vi "ICRA2024测试椭圆分裂0902修改版.vi"() -> ()   [LabVIEW 2018]
doc: "Demonstrates the use of the Network Streams functions to send LED status to the myRIO target."
uses:
  <vilib>/vision/Contour.llb/IMAQ Contour Curve Extraction.ctl
  <vilib>/ErrorRing/Error Ring.xnode
  <vilib>/vision/NI_Vision_Development_Module.lvlib
panel:
  out "数据总":dbl[][](array[numeric])
  out "pitch angle2":dbl[](array[numeric])
  out "pitch angle1":sgl[](array[numeric])
  out "direction angle":sgl[](array[numeric])
  out "磁场ratio":sgl[](array[numeric])
  out "磁场频率":sgl[](array[numeric])
  out "T":i32[](array[numeric])
  out "ratio":dbl[](array[numeric])
  out "长度2":i32[](array[numeric])
  out "宽度":i32[](array[numeric])
  in  "数据记录":bool
  out "ratio":dbl
  out "长度2":i32
  out "宽度":i32
  out "Y Bottom":i32
  out "X Right":i32
  out "Y Top":i32
  out "X Left":i32
  in  "Rectangle 3":T1={"Left"=500, "Top"=800, "Right"=800, "Bottom"=1100}
  in  "Rectangle 2":T1={"Left"=500, "Top"=500, "Right"=800, "Bottom"=600}
  in  "Rectangle":T1={"Left"=500, "Top"=0, "Right"=800, "Bottom"=300}
  in  "Search Rect (entire image)":T2={"Left"=200, "Top"=120, "Right"=2000, "Bottom"=1920, "Rotation"=0.0} {"Rotation" format="%.2f"; "Left" scale=0.0..1024.0; "Right" scale=0.0..1024.0}
  out "长度":dbl
  out "备用的椭圆角度":sgl
  out "Image 9":T3(plugin-control)
  in  "Search Direction":T4(ring)
  in  "Contour Selection":T5(ring)
  in  "Number of Erosion":i32=10
  in  "椭圆磁场开关":bool=TRUE
  out "Image 7":T3(plugin-control)
  out "Ellipse":T6 {"Center"."Y" format="%.2f"; "Center"."X" format="%.2f"}
  out "Image 5":T3(plugin-control)
  in  "Contour Points Settings":T7={"Overlay?"=FALSE, "Color"=16711680, "Width"=1, "Maintain Width?"=TRUE}
  in  "Contour Equation Settings":T7={"Overlay?"=TRUE, "Color"=3381759, "Width"=1, "Maintain Width?"=TRUE}
  out "ROI Descriptor Out":T8 {"Contours"."Type" items=["No Selection", "Point", "Line", "Rectangle", "Oval", "Polygon", "Freehand Region", "Annulus", "Unused2", "Unused3", "Broken Line", "Freehand Line", "Rotated Rectangle"]}
  in  "Curve Extraction":T9={"Extraction Mode"=0, "Edge Threshold"=75, "Edge Filter Size"=1, "Min Length"=25, "Search Step Size"=15, "Max Endpoint Gap"=10, "Subpixel"=TRUE} {"Extraction Mode" items=["Normal", "Uniform Regions"]; "Edge Filter Size" items=["Fine", "Normal", "Contour Tracing"]; "Max Endpoint Gap" min=0; "Search Step Size" min=1 max=255 step=1; "Min Length" min=0; "Edge Threshold" min=1 max=350 step=1}
  out "Image 4":T3(plugin-control)
  out "Image":T3(plugin-control)
  in  "Acquisition Control::Acquisition Frame Rate":dbl=19.50304412841797 min=1.4211589097976685 max=44.94382095336914
  out "Stopped":bool
  in  "Stop (F) 2":bool caption="Stop (F)"
  out "Objects 2":T10(array[cluster]) {"Aspect Ratio" format="%.2f"; "Orientation" format="%.2f"; "Area" format="%.2f"; "Object Center"."Y" format="%.2f"; "Object Center"."X" format="%.2f"}
  in  "Settings 2":T11={"Objects"=0, "Threshold"=128, "Reject Border"=FALSE, "Fill Holes"=FALSE, "Min Object Size"=TRUE, "Min Size"=20000, "Max Object Size"=FALSE, "Max Size"=100, "Show Search Area"=FALSE, "Show Center"=TRUE, "Show Bounding Box"=TRUE} {"Objects" items=["Bright Objects", "Dark Objects"]; "Threshold" min=1 max=999999999 step=1; "Max Size" min=1 max=999999999 step=1; "Min Size" min=1 max=999999999 step=1}
  in  "Range 2":cluster{"Lower value":sgl, "Upper value":sgl}={"Lower value"=0.0, "Upper value"=230.0} {"Upper value" format="%.2f"; "Lower value" format="%.2f"}
  in  "Pause":bool
  out "Array":dbl[](array[numeric])
  in  "Parameter Settings":T12(tab)=enum."Ribbon Oscillating Field" caption="Field Types"
  in  "fg":dbl
  in  "pg":dbl
  in  "dg":dbl
  in  "Ag":dbl
  in  "AoOF":dbl
  in  "fo":sgl
  in  "do":sgl
  in  "oo":sgl
  in  "po":sgl
  in  "cc":sgl
  in  "pc":sgl
  in  "wc":sgl
  in  "dc":sgl
  in  "Ac":dbl
  in  "pr":sgl
  in  "Ar":dbl=8.0
  in  "wr":sgl=18.0
  in  "dr":sgl
  in  "Dis phase step":dbl
  in  "Dis phase frequency (Hz)":dbl
  in  "Dis tumbling frequency (Hz)":dbl
  in  "Dis strength(mT)":dbl
  in  "Swa strength (mT)":dbl
  in  "Swa frequency (Hz)":dbl
  in  "Swa pitch angle (deg)":dbl
  in  "Swa direction angle (deg)":dbl
  in  "Swa ratio":dbl=1.0
  in  "Pitch Angle (rotating around Constant, deg)":dbl
  in  "Ratio (A/C)":sgl=3.0
  in  "Direction Angle (deg)":sgl=90.0
  in  "Pitch Angle (rotating around Origin, deg)":sgl
  in  "Frequency (Hz)":sgl=6.0
  in  "Strength (mT)":dbl=3.0
  in  "Ar 2":dbl=5.0 caption="Ar"
  in  "ratio":sgl=1.0
  in  "运动方向":sgl
  in  "长轴方向":sgl
  in  "wr  2":sgl=8.0
  in  "速度大小":sgl
  out "Angle":dbl
  out "aspect ratio":dbl
  out "时间":i32
  out "Numeric 5":i32
  in  "Stop":bool
  out "error out":errorcluster
  in  "Target IP Address":string="172.22.11.2"
  # "Overview: Magnetic field calculation, and send parameters to myRIO\nInstructions:\n1. Verify the value of Target IP Address. Set Visa resource name.\n2. Ensure RT Main.vi is already running. \n3. Run this VI. Set parameters of magnetic field."
  # "Strength (mT)"
  # "Pitch Angle (deg)"
  # "Direction Angle (deg)"
  # "Frequency (Hz)"
  # "Strength (mT)"
  # "Oscilation Frequency (Hz)"
  # "Oscilation Angle (deg)"
  # "Pitch Angle (deg)"
  # "Direction Angle (deg)"
  # "Strength (mT)"
  # "Frequency (Hz)"
  # "Pitch Angle (deg)"
  # "Direction Angle (deg)"
  # "Conical Angle (deg)"
  # "Strength (mT)"
  # "Frequency (Hz)"
  # "Pitch Angle (deg)"
  # "Direction Angle (deg)"
  # "Strength (mT)"
  # "Tumbling Frequency (Hz)"
  # "Phase Frequency (Hz)"
  # "Phase Step"
  # "Strength (mT)"
  # "Frequency (Hz)"
  # "Pitch Angle (deg)"
  # "Direction Angle (deg)"
  # "Ratio"
  # "Strength (mT)"
  # "Frequency (Hz)"
  # "Ratio (A/C)"
  # "Direction Angle (deg)"
  # "Pitch Angle (rotating around Origin, deg)"
  # "Pitch Angle (rotating around Constant, deg)"
  # "Strength (mT)"
  # "Frequency (Hz)"
  # "Pitch Angle  (deg)"
  # "longaxis"
  # "Direction Angle (deg)"
  # "ratio (l/s)"
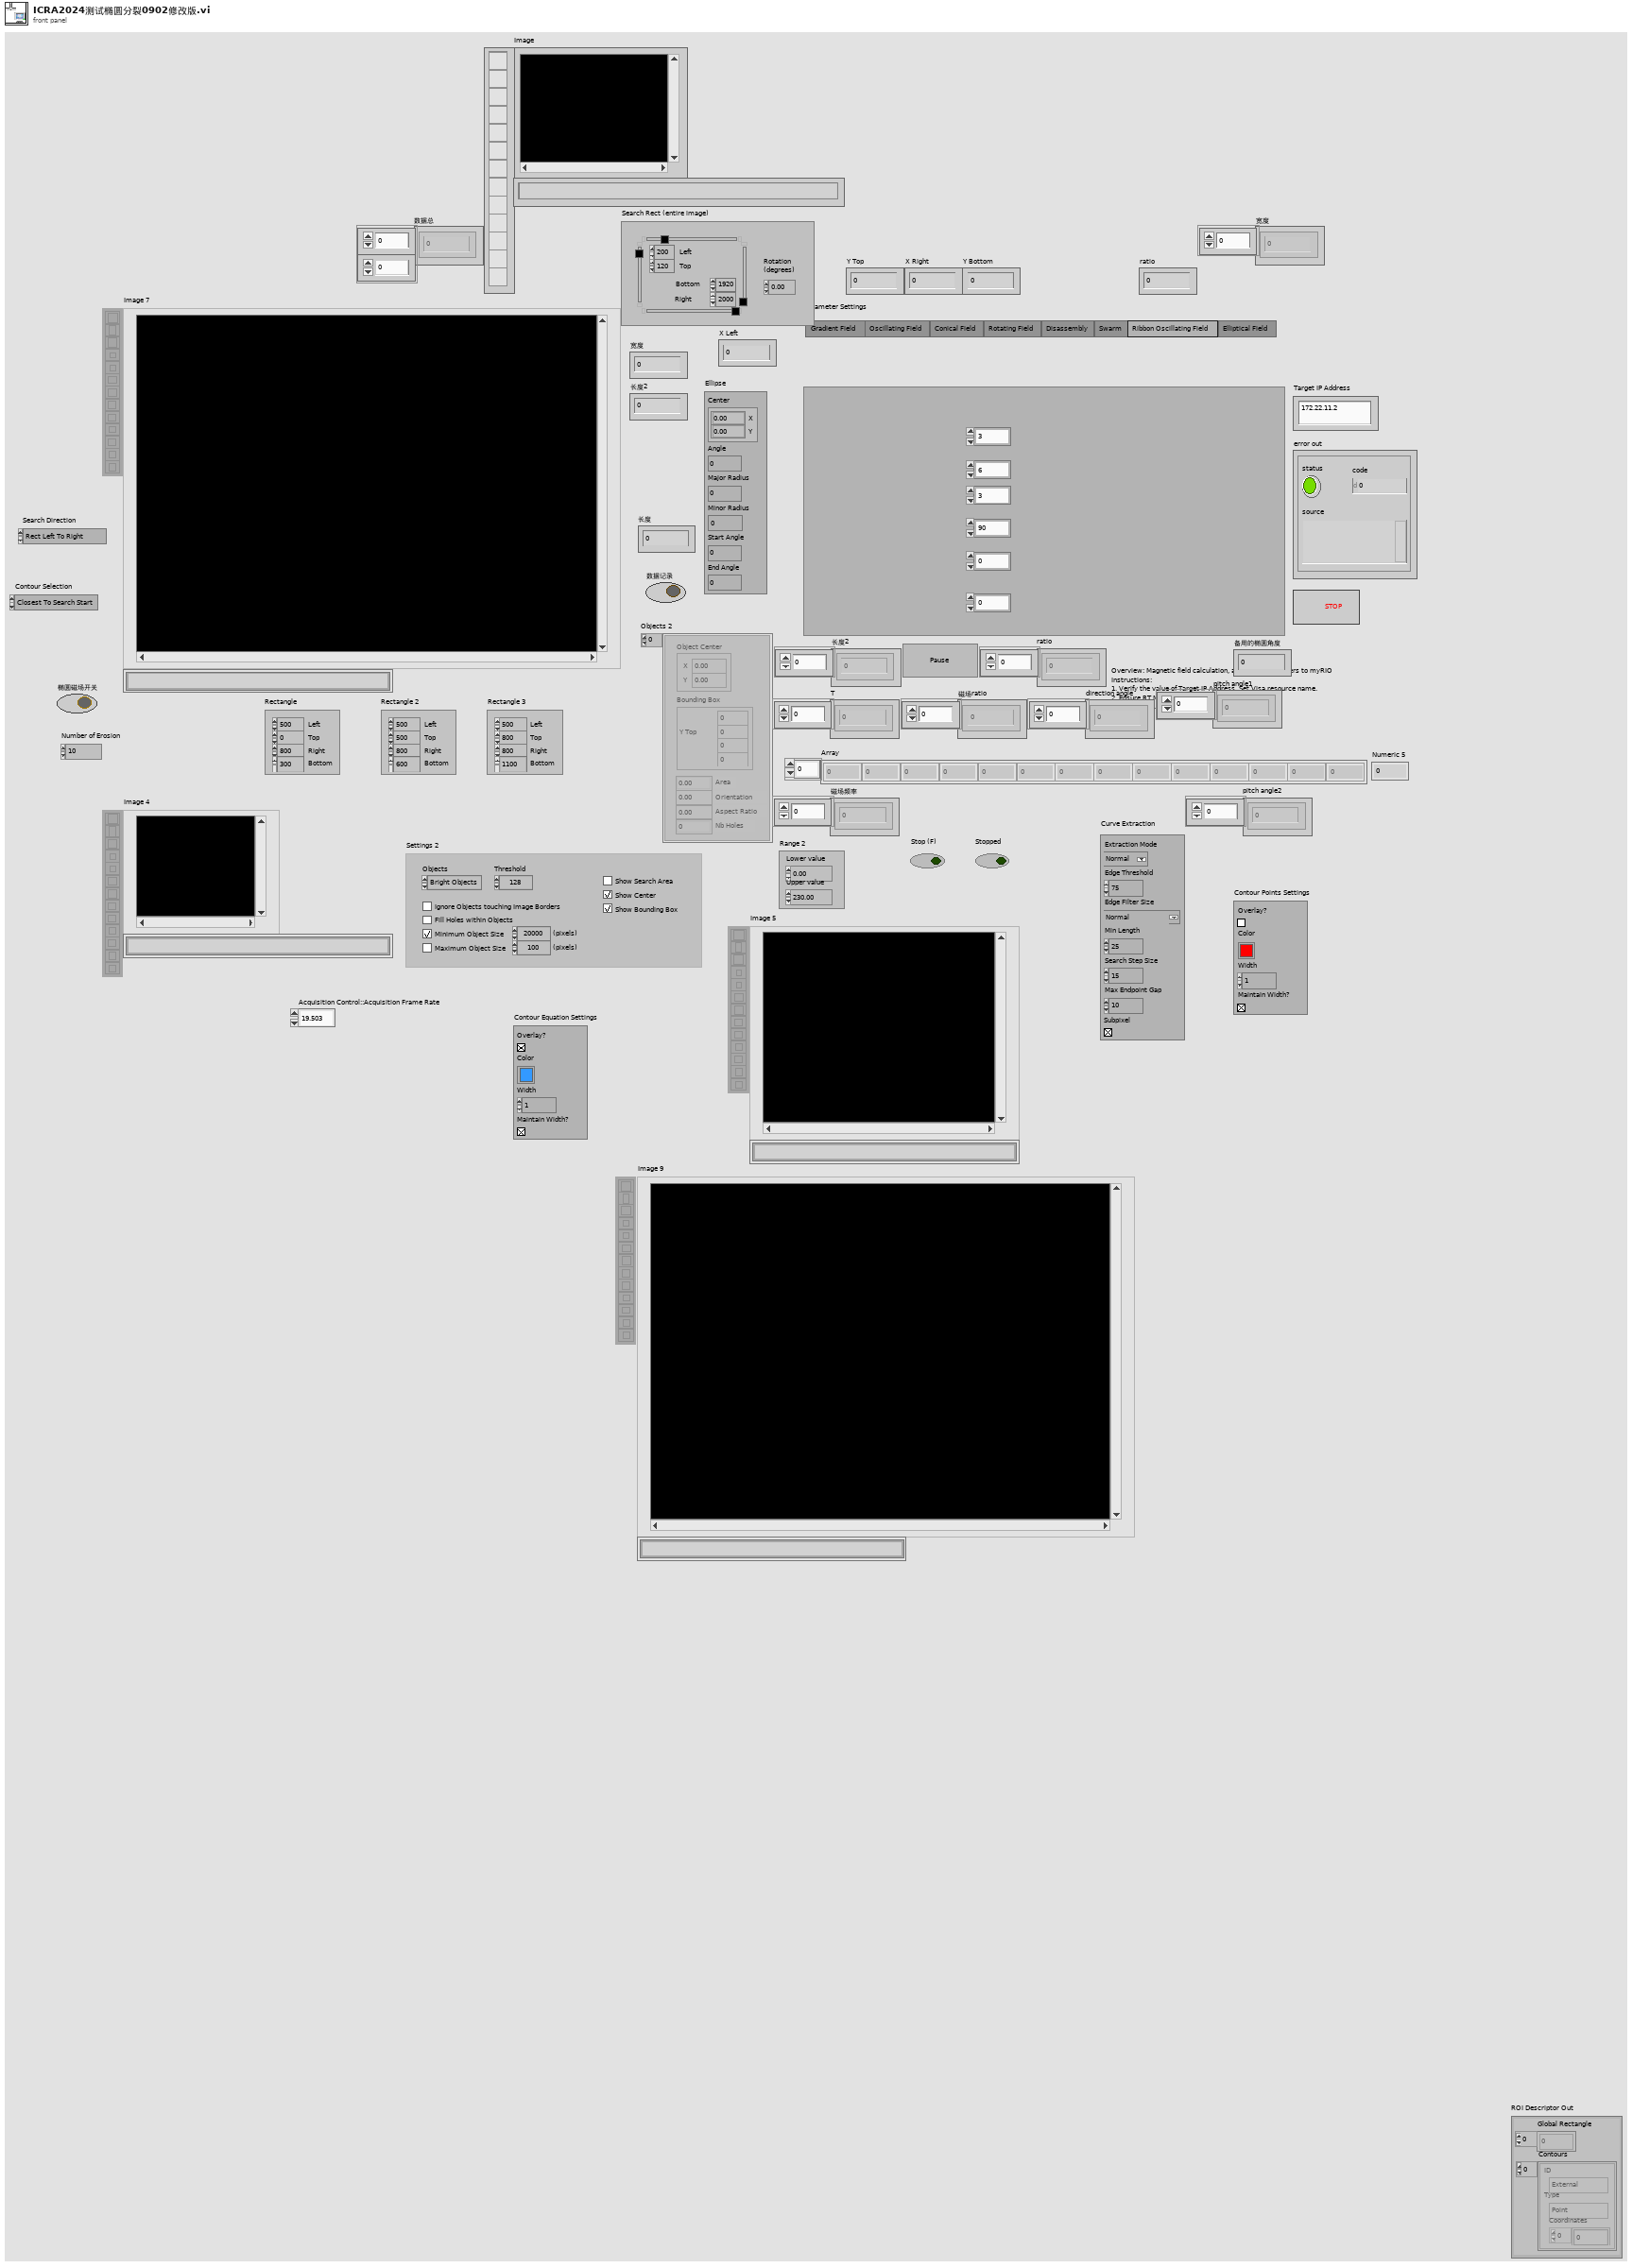
[diagram p1: front panel]
types:
  T1 = cluster{"Left":i32, "Top":i32, "Right":i32, "Bottom":i32}
  T2 = typedef "IMAQ Rectangle" = cluster{"Left":i32, "Top":i32, "Right":i32, "Bottom":i32, "Rotation":dbl}
  T3 = typedef "IMAQ Image.ctl" = refnum<image>
  T4 = enum16{"Rect Left To Right", "Rect Right To Left", "Rect Top To Bottom", "Rect Bottom To Top", "Annulus Inner To Outer", "Annulus Outer To Inner", "Annulus Start Angle To End Angle", "Annulus End Angle To Start Angle"}
  T5 = enum16{"Closest To Search Start", "Maximum Length", "Strongest Mean Gradient Change"}
  T6 = cluster{"Center":cluster{"X":sgl, "Y":sgl}, "Angle":dbl, "Major Radius":dbl, "Minor Radius":dbl, "Start Angle":dbl, "End Angle":dbl}
  T7 = cluster{"Overlay?":bool, "Color":u32, "Width":u32, "Maintain Width?":bool}
  T8 = typedef "ROI Descriptor" = cluster{"Global Rectangle":i32[], "Contours":cluster{"ID":enum32{"External", "Internal"}, "Type":u32, "Coordinates":i32[]}[]}
  T9 = typedef "IMAQ Contour Curve Extraction.ctl" = cluster{"Extraction Mode":u32, "Edge Threshold":i32, "Edge Filter Size":u32, "Min Length":i32, "Search Step Size":i32, "Max Endpoint Gap":i32, "Subpixel":bool}
  T10 = cluster{"Object Center":cluster{"X":sgl, "Y":sgl}, "Bounding Box":cluster{"X Left":i32, "Y Top":i32, "X Right":i32, "Y Bottom":i32}, "Area":sgl, "Orientation":sgl, "Aspect Ratio":sgl, "Nb Holes":i32}[]
  T11 = cluster{"Objects":u16, "Threshold":i32, "Reject Border":bool, "Fill Holes":bool, "Min Object Size":bool, "Min Size":i32, "Max Object Size":bool, "Max Size":i32, "Show Search Area":bool, "Show Center":bool, "Show Bounding Box":bool}
  T12 = enum32{"Gradient Field ", "Oscillating Field", "Conical Field", "Rotating Field", "Disassembly", "Swarm", "Ribbon Oscillating Field", "Elliptical Field"}
  T13 = enum32{"AutoM", "Close", "Dilate", "Erode", "Gradient", "Gradient in", "Gradient out", "HitMiss", "Open", "PClose", "POpen", "Thick", "Thin"}
  T14 = typedef "Image Type" = u32
  T15 = cluster{"Objects[0]":cluster{"Object Center":cluster{"X":sgl, "Y":sgl}, "Bounding Box":cluster{"X Left":i32, "Y Top":i32, "X Right":i32, "Y Bottom":i32}, "Area":sgl, "Orientation":sgl, "Aspect Ratio":sgl, "Nb Holes":i32}, "Objects[1]":cluster{"Object Center":cluster{"X":sgl, "Y":sgl}, "Bounding Box":cluster{"X Left":i32, "Y Top":i32, "X Right":i32, "Y Bottom":i32}, "Area":sgl, "Orientation":sgl, "Aspect Ratio":sgl, "Nb Holes":i32}, "Objects[2]":cluster{"Object Center":cluster{"X":sgl, "Y":sgl}, "Bounding Box":cluster{"X Left":i32, "Y Top":i32, "X Right":i32, "Y Bottom":i32}, "Area":sgl, "Orientation":sgl, "Aspect Ratio":sgl, "Nb Holes":i32}, "Objects[3]":cluster{"Object Center":cluster{"X":sgl, "Y":sgl}, "Bounding Box":cluster{"X Left":i32, "Y Top":i32, "X Right":i32, "Y Bottom":i32}, "Area":sgl, "Orientation":sgl, "Aspect Ratio":sgl, "Nb Holes":i32}, "Objects[4]":cluster{"Object Center":cluster{"X":sgl, "Y":sgl}, "Bounding Box":cluster{"X Left":i32, "Y Top":i32, "X Right":i32, "Y Bottom":i32}, "Area":sgl, "Orientation":sgl, "Aspect Ratio":sgl, "Nb Holes":i32}, "Objects[5]":cluster{"Object Center":cluster{"X":sgl, "Y":sgl}, "Bounding Box":cluster{"X Left":i32, "Y Top":i32, "X Right":i32, "Y Bottom":i32}, "Area":sgl, "Orientation":sgl, "Aspect Ratio":sgl, "Nb Holes":i32}, "Objects[6]":cluster{"Object Center":cluster{"X":sgl, "Y":sgl}, "Bounding Box":cluster{"X Left":i32, "Y Top":i32, "X Right":i32, "Y Bottom":i32}, "Area":sgl, "Orientation":sgl, "Aspect Ratio":sgl, "Nb Holes":i32}, "Objects[7]":cluster{"Object Center":cluster{"X":sgl, "Y":sgl}, "Bounding Box":cluster{"X Left":i32, "Y Top":i32, "X Right":i32, "Y Bottom":i32}, "Area":sgl, "Orientation":sgl, "Aspect Ratio":sgl, "Nb Holes":i32}, "Objects[8]":cluster{"Object Center":cluster{"X":sgl, "Y":sgl}, "Bounding Box":cluster{"X Left":i32, "Y Top":i32, "X Right":i32, "Y Bottom":i32}, "Area":sgl, "Orientation":sgl, "Aspect Ratio":sgl, "Nb Holes":i32}}
  T16 = cluster{"Object Center":cluster{"X":sgl, "Y":sgl}, "Bounding Box":cluster{"X Left":i32, "Y Top":i32, "X Right":i32, "Y Bottom":i32}, "Area":sgl, "Orientation":sgl, "Aspect Ratio":sgl, "Nb Holes":i32}
  T17 = cluster{"X Left":i32, "Y Top":i32, "X Right":i32, "Y Bottom":i32}
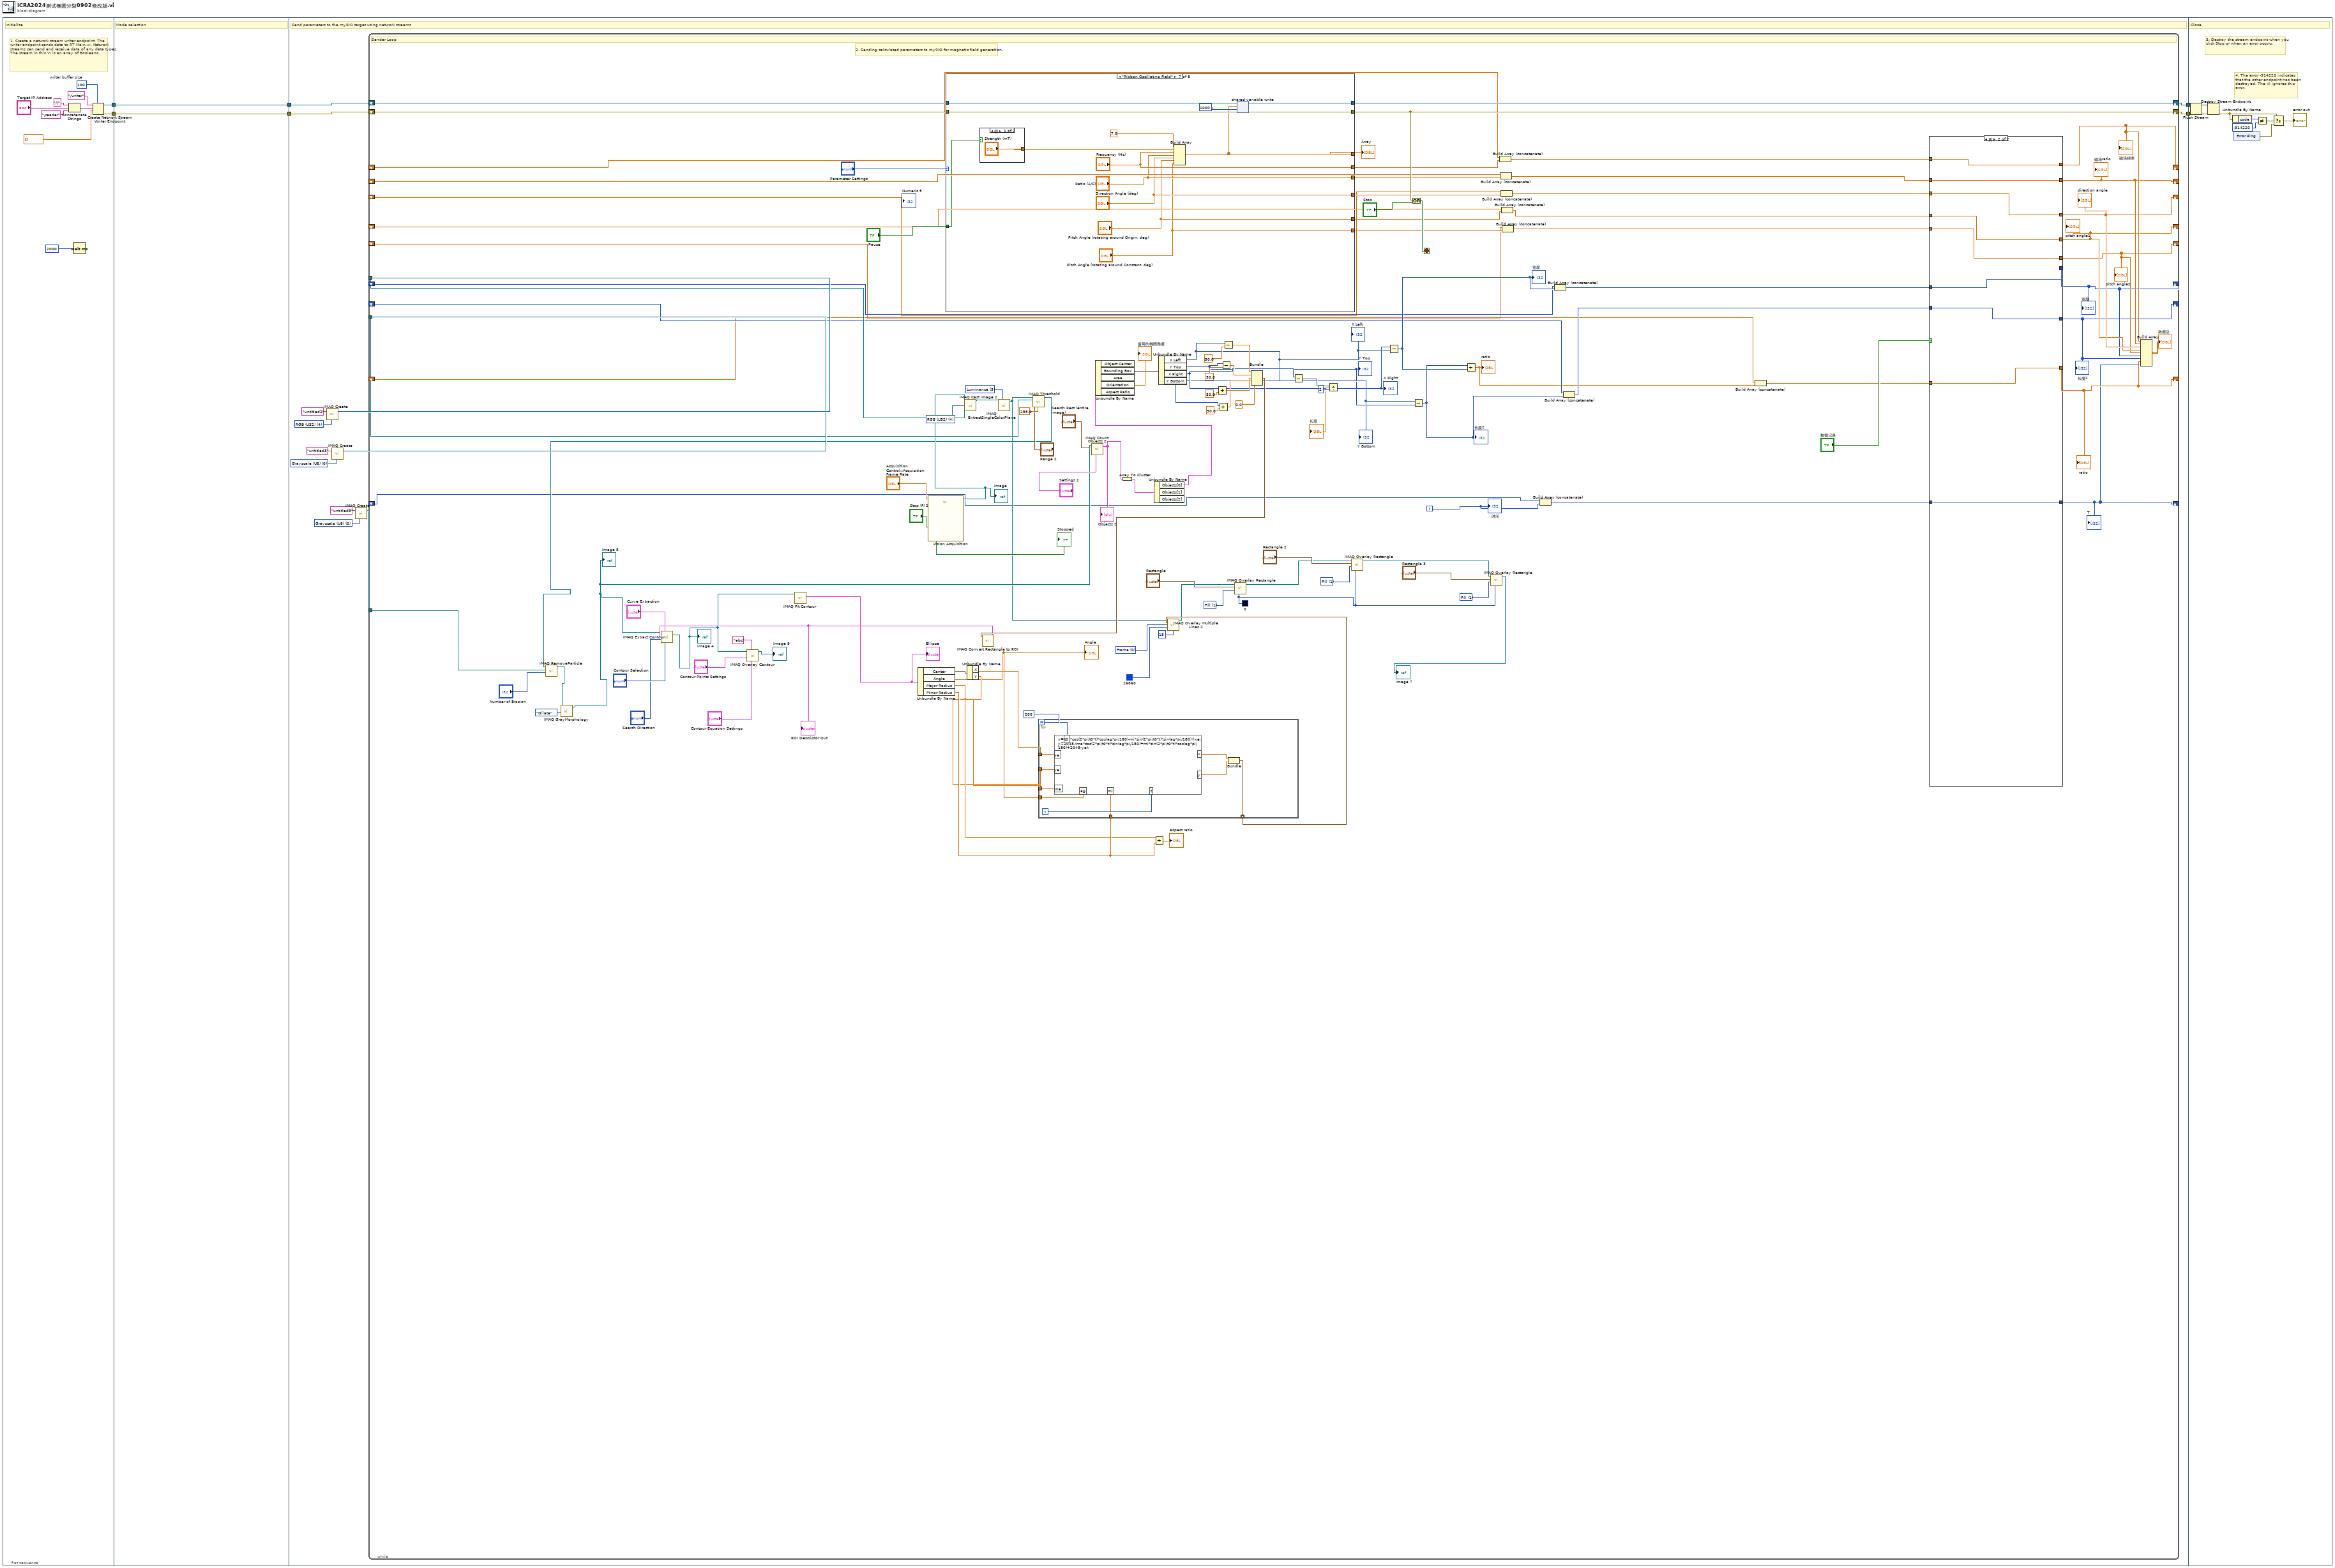
[diagram p0: block diagram]
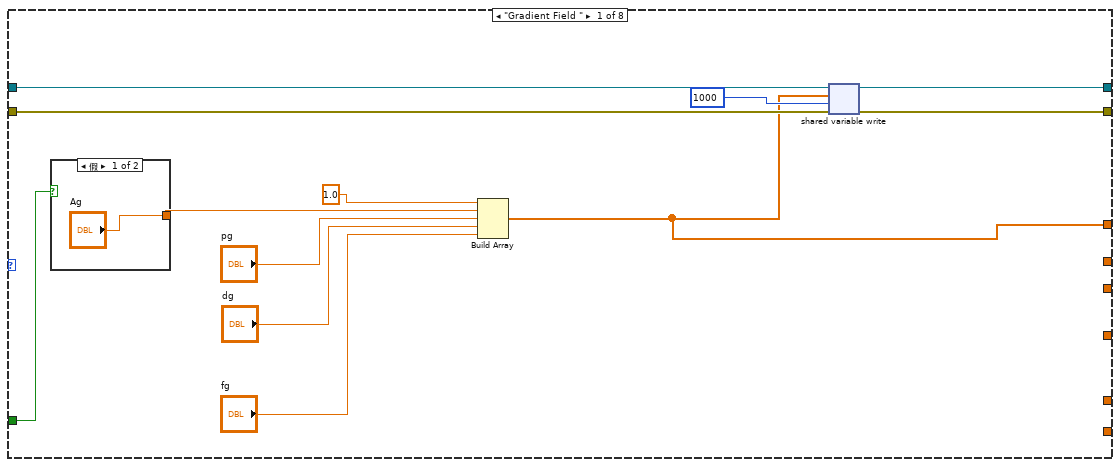
[diagram p3: hidden frame]
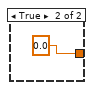
[diagram p4: hidden frame]
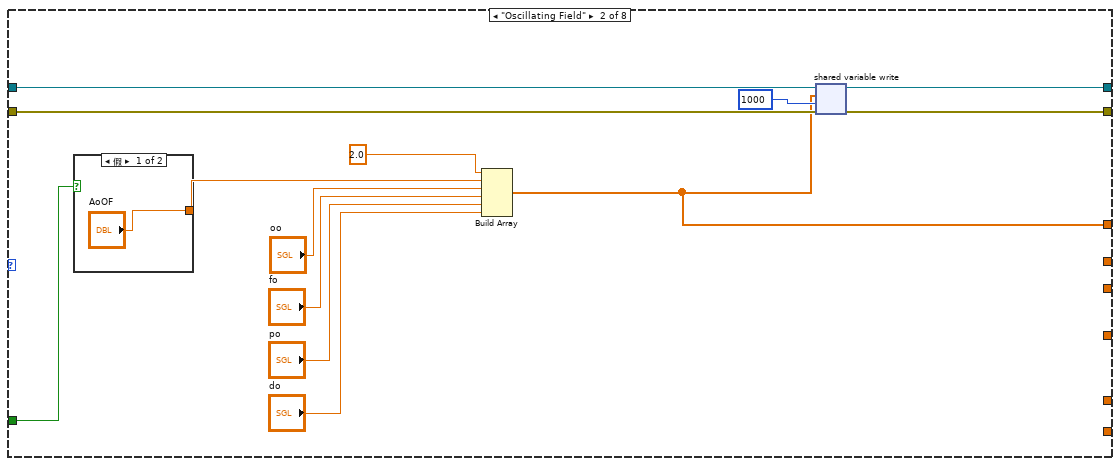
[diagram p5: hidden frame]
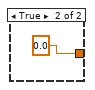
[diagram p6: hidden frame]
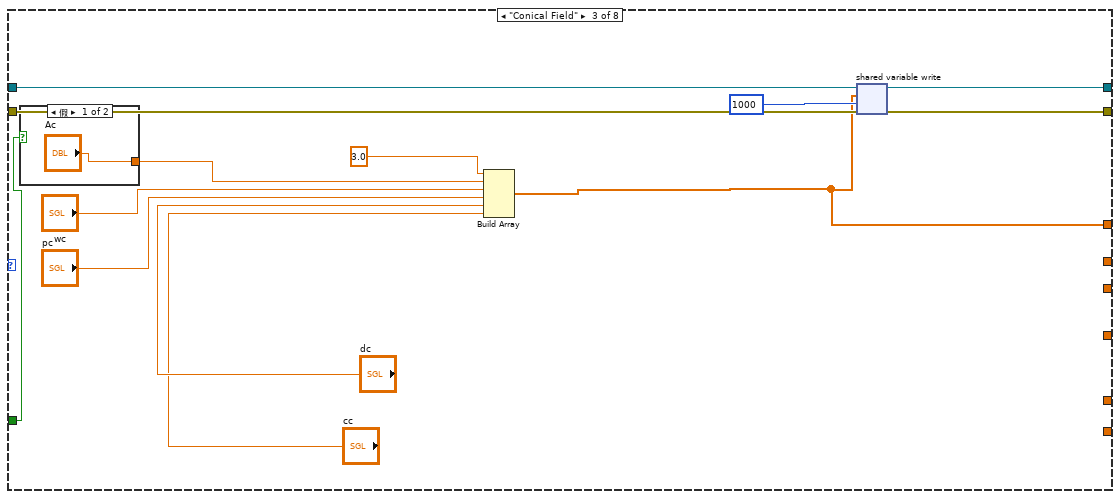
[diagram p7: hidden frame]
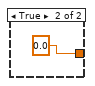
[diagram p8: hidden frame]
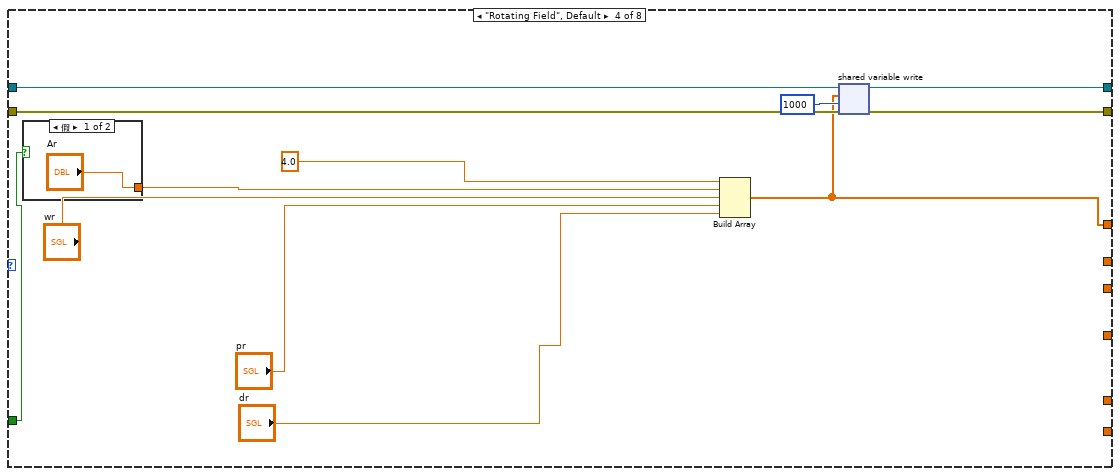
[diagram p9: hidden frame]
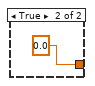
[diagram p10: hidden frame]
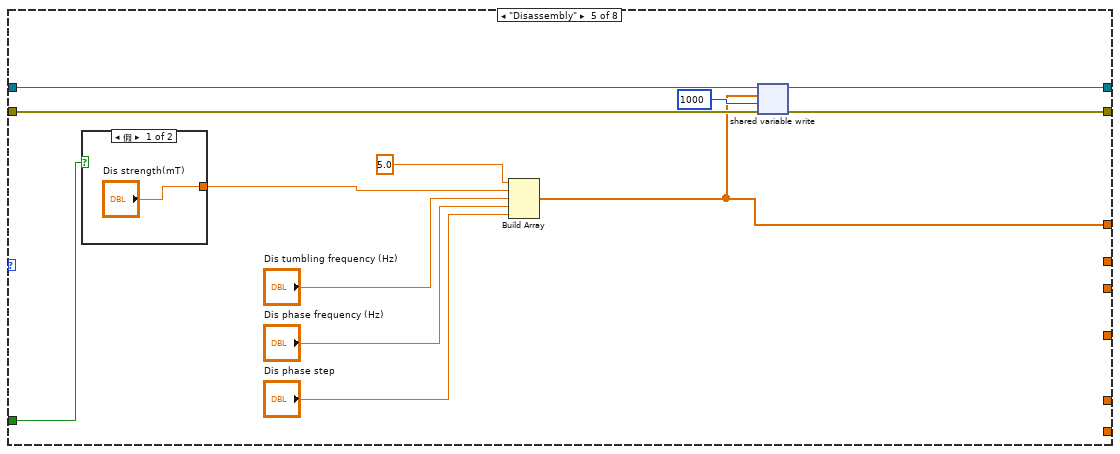
[diagram p11: hidden frame]
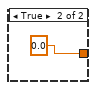
[diagram p12: hidden frame]
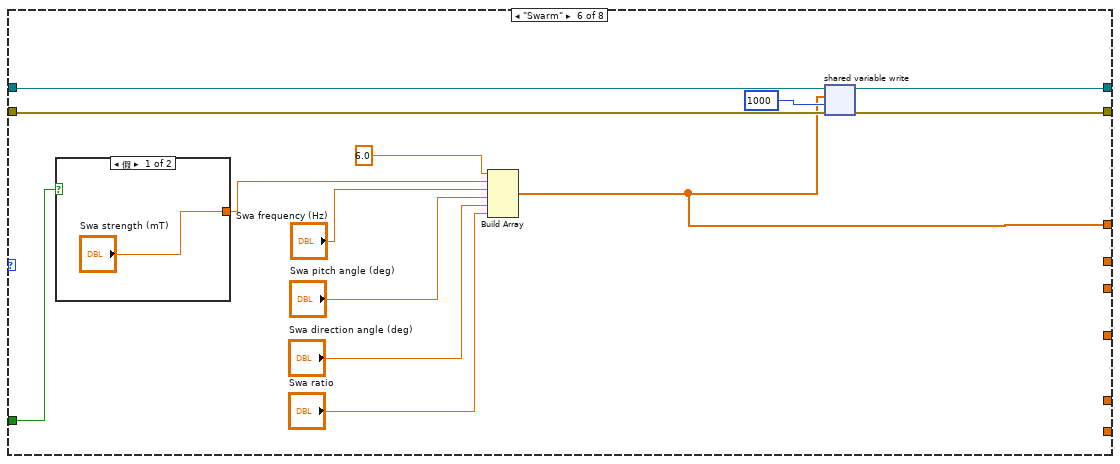
[diagram p13: hidden frame]
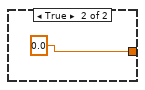
[diagram p14: hidden frame]
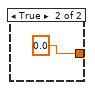
[diagram p15: hidden frame]
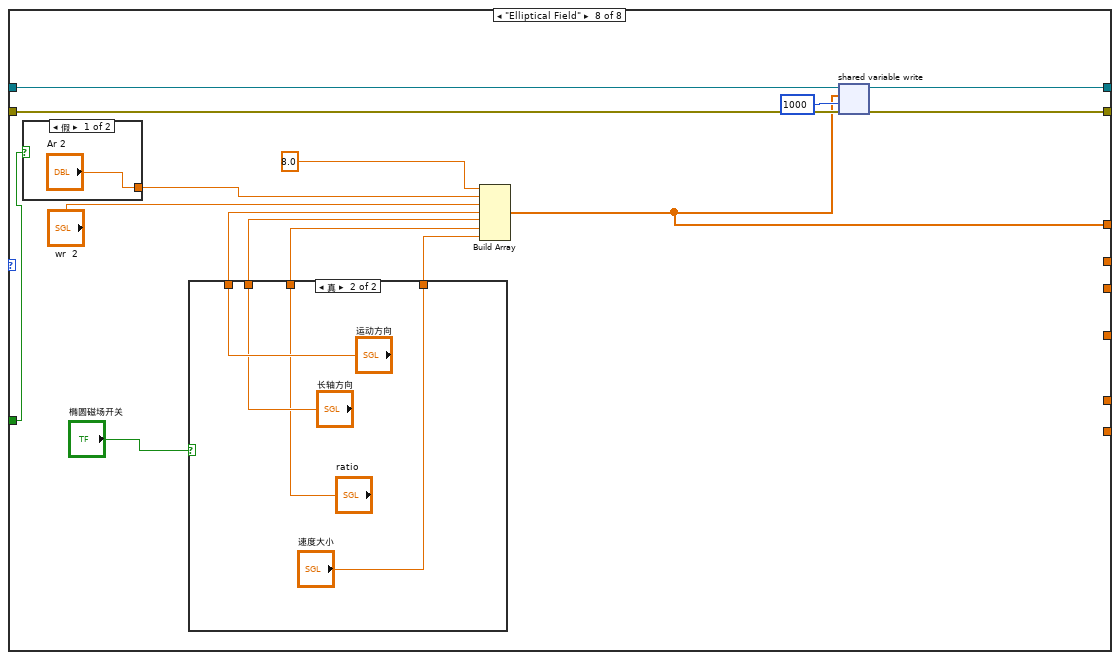
[diagram p16: hidden frame]
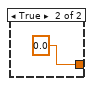
[diagram p18: hidden frame]
diagram:
  n1 = flat-sequence {
    tunnel: [w11] -> w2
    tunnel: [w10] -> w1
    tunnel: [w18] -> w4
    tunnel: [w17] -> w3
    tunnel: w1 -> [w17]
    tunnel: w2 -> [w18]
    tunnel: [w29] -> w6
    tunnel: w4 -> [w31]
    tunnel: [w28] -> w5
    tunnel: w3 -> [w30]
    tunnel: w6 -> [w306]
    tunnel: w5 -> [w303]
    frame #0 {
      w9 = 100  # writer buffer size
      # "1. Create a network stream writer endpoint. The writer endpoint sends data to RT Main.vi. Network streams can send and receive data of any data types. The stream in this VI is an array of Booleans."
      # "Initialize"
      n2 = Concatenate Strings("//", "Target IP Address", "/reader") -> (w16:string)
      n3 = Wait (ms)(milliseconds to wait=2000) -> ()  [unwired: 1 out]
      n4 = Create Network Stream Writer Endpoint(7:w9, 9:dbl[] [], 10:w16, 11:"/writer" ("reader name")) -> (0:w10:errorcluster, 3:w11:refnum<k21>)  [unwired: 3 in]
    }
    frame #1 {
      # "Mode selection"
    }
    frame #2 {
      w20 = T14 0 items=["Grayscale (U8)", "Grayscale (I16)", "Grayscale (SGL)", "Complex (CSG)", "RGB (U32)", "HSL (U32)", "RGB (U64)", "Grayscale (U16)"] ("Image Type")
      w24 = T14 0 items=["Grayscale (U8)", "Grayscale (I16)", "Grayscale (SGL)", "Complex (CSG)", "RGB (U32)", "HSL (U32)", "RGB (U64)", "Grayscale (U16)"] ("Image Type")
      w26 = T14 4 items=["Grayscale (U8)", "Grayscale (I16)", "Grayscale (SGL)", "Complex (CSG)", "RGB (U32)", "HSL (U32)", "RGB (U64)", "Grayscale (U16)"] ("Image Type")
      # "Send parameters to the myRIO target using network streams"
      n5 = call "IMAQ Create"("Image Name"="untitled2", "Image Type"=w26) -> ("New Image"=w23:T3)  [unwired: 3 in, 1 out]
      n6 = call "IMAQ Create"("Image Name"="untitled3", "Image Type"=w24) -> ("New Image"=w22:T3)  [unwired: 3 in, 1 out]
      n7 = call "IMAQ Create"("Image Name"="untitled3", "Image Type"=w20) -> ("New Image"=w19:T3)  [unwired: 3 in, 1 out]
      n8 = while {
        shift-right: [w149] -> w28
        shift-left: w30 -> [w151]
        shift-right: [w150] -> w29
        shift-left: w31 -> [w152]
        tunnel: w22 -> [w140]
        tunnel: w23 -> [w135]
        tunnel: w19 -> [w105]
        shift-right: [w36] -> _
        shift-left: _ -> [w66]
        shift-right: [w35] -> _
        shift-left: _ -> [w63]
        shift-right: [w34] -> _
        shift-left: _ -> [w60]
        shift-right: [w33] -> _
        shift-left: _ -> [w57]
        shift-right: [w41] -> _
        shift-left: _ -> [w54]
        shift-right: [w40] -> _
        shift-left: _ -> [w51]
        shift-right: [w39] -> _
        shift-left: _ -> [w48]
        shift-right: [w38] -> _
        shift-left: _ -> [w45]
        shift-right: [w37] -> _
        shift-left: _ -> [w42]
        i -> [w59]
        stop <- w139 stop-if-true
        w74 = u32 0 ("Color")
        w77 = u32 1 items=["Frame", "Fill", "Highlight"] ("Drawing Mode (Frame)")
        w79 = u32 1 items=["Frame", "Fill", "Highlight"] ("Drawing Mode (Frame)")
        w84 = u32 1 items=["Frame", "Fill", "Highlight"] ("Drawing Mode (Frame)")
        w122 = u32 0 items=["Frame", "Fill"] ("Drawing Mode (Frame)")
        w134 = T14 4 items=["Grayscale (U8)", "Grayscale (I16)", "Grayscale (SGL)", "Complex (CSG)", "RGB (U32)", "HSL (U32)", "RGB (U64)", "Grayscale (U16)"] ("Image Type")
        w145 = 5 items=["Red", "Green", "Blue", "Hue", "Saturation", "Luminance", "Value", "Intensity"] ("Color Plane")
        # "2. Sending calculated parameters to myRIO for magnetic field generation."
        # "Sender Loop"
        n9 = call "Vision Acquisition"("Acquisition Control::Acquisition Frame Rate"="Acquisition Control::Acquisition Frame Rate", "Stop (F)"="Stop (F) 2") -> ("Image Out"=w133:T3, "Stopped"=→"Stopped":bool)  [unwired: 23 in, 1 out]
        "Image" <- w133
        n10 = case shown="\"Ribbon Oscillating Field\"" "Parameter Settings" {
          tunnel: w152 -> [w183 w198 w213 w227 w241 w255 w273 w289]
          tunnel: w151 -> [w180 w197 w212 w226 w239 w254 w271 w288]
          tunnel: [w182 w196 w210 w225 w240 w253 w272 w287] -> w150
          tunnel: [w181 w195 w211 w224 w238 w252 w270 w286] -> w149
          tunnel: [w176 w189 w204 w219 w232 w247 w268 w281] -> w148
          tunnel: "Pause" -> [w174 w187 w202 w217 w231 w246 w266 w279]
          tunnel: [_ _ _ _ _ _ "Frequency (Hz)" _] -> w56
          tunnel: [_ _ _ _ _ _ "Ratio (A/C)" _] -> w53
          tunnel: [_ _ _ _ _ _ "Direction Angle (deg)" _] -> w50
          tunnel: [_ _ _ _ _ _ "Pitch Angle (rotating around Origin, deg)" _] -> w47
          tunnel: [_ _ _ _ _ _ "Pitch Angle (rotating around Constant, deg)" _] -> w44
          frame "Gradient Field " {
            n11 = case shown="假" w174 {
              tunnel: ["Ag" 0.0] -> w175
              frame False {
              }
              frame True {
              }
            }
            n12 = Build Array(1.0, w175, "pg", "dg", "fg") -> (w176:dbl[])
            n13 = shared-variable-write(w183, w180, w176, 1000 ("timeout ms (-1)")) -> (w182:refnum<k21>, w181:errorcluster)  [unwired: 1 out]
          }
          frame "Oscillating Field" {
            n14 = case shown="假" w187 {
              tunnel: ["AoOF" 0.0] -> w188
              frame False {
              }
              frame True {
              }
            }
            n15 = Build Array(2.0, w188, "oo", "fo", "po", "do") -> (w189:dbl[])
            n16 = shared-variable-write(w198, w197, w189, 1000 ("timeout ms (-1)")) -> (w196:refnum<k21>, w195:errorcluster)  [unwired: 1 out]
          }
          frame "Conical Field" {
            # "FG"
            n17 = case shown="假" w202 {
              tunnel: ["Ac" 0.0] -> w203
              frame False {
              }
              frame True {
              }
            }
            n18 = Build Array(3.0, w203, "wc", "pc", "dc", "cc") -> (w204:dbl[])
            n19 = shared-variable-write(w213, w212, w204, 1000 ("timeout ms (-1)")) -> (w210:refnum<k21>, w211:errorcluster)  [unwired: 1 out]
          }
          frame "Rotating Field", Default {
            n20 = case shown="假" w217 {
              tunnel: ["Ar" 0.0] -> w218
              frame False {
              }
              frame True {
              }
            }
            n21 = Build Array(4.0, w218, "wr", "pr", "dr") -> (w219:dbl[])
            n22 = shared-variable-write(w227, w226, w219, 1000 ("timeout ms (-1)")) -> (w225:refnum<k21>, w224:errorcluster)  [unwired: 1 out]
          }
          frame "Disassembly" {
            n23 = case shown="假" w231 {
              tunnel: ["Dis strength(mT)" 0.0] -> w236
              frame False {
              }
              frame True {
              }
            }
            n24 = Build Array(5.0, w236, "Dis tumbling frequency (Hz)", "Dis phase frequency (Hz)", "Dis phase step") -> (w232:dbl[])
            n25 = shared-variable-write(w241, w239, w232, 1000 ("timeout ms (-1)")) -> (w240:refnum<k21>, w238:errorcluster)  [unwired: 1 out]
          }
          frame "Swarm" {
            n26 = case shown="假" w246 {
              tunnel: ["Swa strength (mT)" 0.0] -> w245
              frame False {
              }
              frame True {
              }
            }
            n27 = Build Array(6.0, w245, "Swa frequency (Hz)", "Swa pitch angle (deg)", "Swa direction angle (deg)", "Swa ratio") -> (w247:dbl[])
            n28 = shared-variable-write(w255, w254, w247, 1000 ("timeout ms (-1)")) -> (w253:refnum<k21>, w252:errorcluster)  [unwired: 1 out]
          }
          frame "Ribbon Oscillating Field" {
            n29 = case shown="假" w266 {
              tunnel: ["Strength (mT)" 0.0] -> w265
              frame False {
              }
              frame True {
              }
            }
            n30 = Build Array(7.0, w265, "Frequency (Hz)", "Ratio (A/C)", "Direction Angle (deg)", "Pitch Angle (rotating around Origin, deg)", "Pitch Angle (rotating around Constant, deg)") -> (w268:dbl[])
            n31 = shared-variable-write(w273, w271, w268, 1000 ("timeout ms (-1)")) -> (w272:refnum<k21>, w270:errorcluster)  [unwired: 1 out]
          }
          frame "Elliptical Field" {
            n32 = case shown="假" w279 {
              tunnel: ["Ar 2" 0.0] -> w280
              frame False {
              }
              frame True {
              }
            }
            n33 = case shown="真" "椭圆磁场开关" {
              tunnel: [_ "运动方向"] -> w284
              tunnel: [_ "长轴方向"] -> w283
              tunnel: [_ "ratio"] -> w278
              tunnel: [_ "速度大小"] -> w277
              frame False {
              }
              frame True {
              }
            }
            n34 = Build Array(8.0, w280, "wr  2", w284, w283, w278, w277) -> (w281:dbl[])
            n35 = shared-variable-write(w289, w288, w281, 1000 ("timeout ms (-1)")) -> (w287:refnum<k21>, w286:errorcluster)  [unwired: 1 out]
          }
        }
        "Array" <- w148
        n36 = call "IMAQ Cast Image 2"("Image Src"=w133, "Image Dst"=w135, "Image Type"=w134) -> ("Image Dst Out"=w136:T3)  [unwired: 11 in, 1 out]
        n37 = call "IMAQ ExtractSingleColorPlane"("Color Plane"=w145, "Image Src"=w136) -> ("Image Dst Out"=w97:T3)  [unwired: 8 in, 1 out]
        n38 = call "IMAQ Threshold"("Replace Value"=sgl 255.0, "Range"="Range 2", "Image Dst"=w140, "Image Src"=w97) -> ("Image Dst Out"=w106:T3)  [unwired: 6 in, 1 out]
        n39 = call "IMAQ RemoveParticle"("Number of Erosion"="Number of Erosion", "Image Dst"=w105, "Image Src"=w106) -> ("Image Dst Out"=w101:T3)  [unwired: 7 in, 1 out]
        n40 = call "IMAQ GrayMorphology"("Operation"=T13."Dilate", "Image Src"=w101) -> ("Image Dst Out"=w98:T3)  [unwired: 8 in, 1 out]
        "Image 5" <- w98
        n41 = call "IMAQ Count Objects 2"("Settings"="Settings 2", "Search Rect (entire image)"="Search Rect (entire image)", "Image"=w98) -> ("Objects"=w141:T10)  [unwired: 4 in, 4 out]
        "Objects 2" <- w141
        n42 = Array To Cluster(array=w141) -> (cluster=w108:T15)
        n43 = Unbundle By Name(w108) -> ("Objects[0]"=w107:T16)  [unwired: 2 out]
        n44 = Unbundle By Name(w107) -> ("Bounding Box"=w121:T17, "Orientation"=→"备用的椭圆角度":sgl)  [unwired: 3 out]
        n45 = Unbundle By Name(w121) -> ("X Left"=w72:i32, "Y Top"=w70:i32, "X Right"=w73:i32, "Y Bottom"=w71:i32)
        "X Left" <- w72
        "Y Top" <- w70
        "X Right" <- w73
        "Y Bottom" <- w71
        n46 = Add(x=w73, y=50.0) -> (x+y=w114:dbl)
        n47 = Add(x=w71, y=50.0) -> (x+y=w113:dbl)
        n48 = Subtract(x=w70, y=50.0) -> (x-y=w115:dbl)
        n49 = Subtract(x=w72, y=50.0) -> (x-y=w116:dbl)
        n50 = Bundle(w116, w115, w114, w113, 0.0) -> (w111:cluster{dbl, dbl, dbl, dbl, dbl})  [unwired: 1 in]
        n51 = call "IMAQ Convert Rectangle to ROI"("Rectangle"=w111) -> ("ROI Descriptor"=w110:T8)  [unwired: 8 in, 1 out]
        "ROI Descriptor Out" <- w110
        n52 = call "IMAQ Extract Contour"("Source Image"=w98, "Curve Extraction"="Curve Extraction", "ROI Descriptor"=w110, "Search Direction"="Search Direction", "Contour Selection"="Contour Selection") -> ("Contour Image Out"=w128:T3)  [unwired: 6 in, 4 out]
        "Image 4" <- w128
        n53 = call "IMAQ Overlay Contour"("Contour Equation Settings"="Contour Equation Settings", "Group"="abc", "Contour Points Settings"="Contour Points Settings", "Image"=w128) -> ("Image Out"=→"Image 9":T3)  [unwired: 6 in, 1 out]
        n54 = call-poly "IMAQ Fit Contour"("Contour Image"=w128) -> ("Ellipse"=w126:T6)  [unwired: 8 in, 2 out]
        "Ellipse" <- w126
        n55 = Unbundle By Name(w126) -> ("Center"=w127:cluster{"X":sgl, "Y":sgl}, "Angle"=w92:dbl, "Major Radius"=w95:dbl, "Minor Radius"=w96:dbl)
        "Angle" <- w92
        n56 = Unbundle By Name(w127) -> ("X"=w94:sgl, "Y"=w93:sgl)
        n57 = for {
          N: 200 -> [w168]
          tunnel: [w169] -> w109 mode=indexing
          tunnel: w94 -> [w167]
          tunnel: w93 -> [w166]
          tunnel: w95 -> [w165]
          tunnel: w92 -> [w164]
          tunnel: w96 -> [w163]
          i -> [w170]
          n58 = formula code="x=ma*cos(2*pi/t0*t)*cos(ag*pi/180)-mi*sin(2*pi/t0*t)*sin(ag*pi/180)+xe;\ny=2048-(ma*cos(2*pi/t0*t)*sin(ag*pi/180)+mi*sin(2*pi/t0*t)*cos(ag*pi/180)+2048-ye);"("xe"=w167, "ye"=w166, "ma"=w165, "ag"=w164, "mi"=w163, "t"=w170, "t0"=w168) -> ("x"=w172:dbl, "y"=w171:dbl)
          n59 = Bundle("x"=w172, "y"=w171) -> (w169:cluster{"x":dbl, "y":dbl})  [unwired: 1 in]
        }
        n60 = Divide(x=w95, y=w96) -> (x/y=→"aspect ratio":dbl)
        n61 = call "IMAQ Overlay Multiple Lines 2"("Image"=w97, "Line End Points"=w109, "Drawing Mode (Frame)"=w122, "Color"=u32 16860, "Width"=u32 15) -> ("Image Out"=w82:T3)  [unwired: 9 in, 1 out]
        n62 = call "IMAQ Overlay Rectangle"("Color"=w74, "Drawing Mode (Frame)"=w84, "Rectangle"="Rectangle", "Image"=w82) -> ("Image Out"=w80:T3)  [unwired: 6 in, 1 out]
        n63 = Subtract(x=w73, y=w72) -> (x-y=w88:i32)
        n64 = Divide(x=w88, y=2) -> (x/y=→"长度":dbl)
        n65 = call "IMAQ Overlay Rectangle"("Color"=w74, "Drawing Mode (Frame)"=w79, "Rectangle"="Rectangle 2", "Image"=w80) -> ("Image Out"=w76:T3)  [unwired: 6 in, 1 out]
        n66 = Subtract(x=w73, y=w72) -> (x-y=w68:i32)
        "宽度" <- w68
        n67 = Or(x=w149, y="Stop") -> (x .or. y?=w139:bool)
        n68 = Subtract(x=w71, y=w70) -> (x-y=w65:i32)
        "长度2" <- w65
        n69 = Divide(x=w65, y=w68) -> (x/y=w62:dbl)
        "ratio" <- w62
        n70 = call "IMAQ Overlay Rectangle"("Color"=w74, "Drawing Mode (Frame)"=w77, "Rectangle"="Rectangle 3", "Image"=w76) -> ("Image Out"=→"Image 7":T3)  [unwired: 6 in, 1 out]
        n71 = Build Array (concatenate)(w54, w56) -> (w55:sgl[])
        n72 = Build Array (concatenate)(w51, w53) -> (w52:sgl[])
        n73 = Build Array (concatenate)(w48, w50) -> (w49:sgl[])
        n74 = Build Array (concatenate)(w45, w47) -> (w46:sgl[])
        n75 = Build Array (concatenate)(w42, w44) -> (w43:dbl[])
        n76 = Build Array (concatenate)(w57, w59) -> (w58:i32[])
        n77 = Build Array (concatenate)(w66, w68) -> (w67:i32[])
        n78 = Build Array (concatenate)(w63, w65) -> (w64:i32[])
        n79 = Build Array (concatenate)(w60, w62) -> (w61:dbl[])
        n80 = case shown="真" "数据记录" {
          tunnel: [_ w162] -> w36
          tunnel: w67 -> [_ w162]
          tunnel: [_ w161] -> w35
          tunnel: w64 -> [_ w161]
          tunnel: [_ w160] -> w34
          tunnel: w61 -> [_ w160]
          tunnel: w58 -> [_ w159]
          tunnel: [_ w159] -> w33
          tunnel: [_ w158] -> w41
          tunnel: w55 -> [_ w158]
          tunnel: [_ w157] -> w40
          tunnel: w52 -> [_ w157]
          tunnel: [_ w156] -> w39
          tunnel: w49 -> [_ w156]
          tunnel: [_ w155] -> w38
          tunnel: w46 -> [_ w155]
          tunnel: [_ w154] -> w37
          tunnel: w43 -> [_ w154]
          frame False {
          }
          frame True {
          }
        }
        "宽度" <- w36
        "长度2" <- w35
        "ratio" <- w34
        "T" <- w33
        "磁场频率" <- w41
        "磁场ratio" <- w40
        "direction angle" <- w39
        "pitch angle1" <- w38
        "pitch angle2" <- w37
        n81 = Build Array(w41, w40, w39, w38, w37, w36, w35, w34, w33) -> (→"数据总":dbl[][])
        "时间" <- w59
      }
    }
    frame #3 {
      # "4. The error -314220 indicates that the other endpoint has been destroyed. The VI ignores this error."
      # "3. Destroy the stream endpoint when you click Stop or when an error occurs."
      # "Close"
      n82 = Flush Stream(8:w303, 11:w306) -> (0:w304:errorcluster, 3:w305:refnum<k21>)  [unwired: 2 in, 1 out]
      n83 = Destroy Stream Endpoint(8:w304, 11:w305) -> (0:w298:errorcluster)
      n84 = Unbundle By Name(w298) -> ("code"=w302:i32)
      n85 = xnode "Error Ring"() -> ("错误输出"=w299:errorcluster)
      n86 = Not Equal?(x=w302, y=-314220) -> (x != y?=w300:bool)
      n87 = Select(t=w298, s=w300, f=w299) -> (s? t:f=→"error out":errorcluster)
    }
  }
